vi "Method 5.vi"(11 "Test Interface in":refnum<class "Test Interface.lvclass">) -> (3 "Test Interface out":refnum<class "Test Interface.lvclass">)   [LabVIEW 2023, in "Test Interface.lvlib" / "Test Interface.lvclass"]
doc: "My Method Description"
uses:
  Test Interface.lvclass
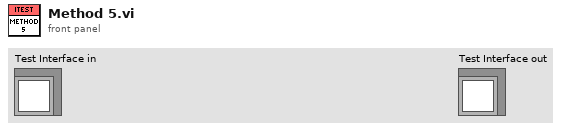
[diagram p1: front panel]
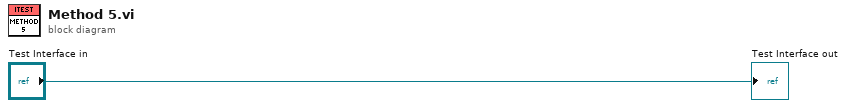
[diagram p0: block diagram]
diagram:
  "Test Interface out" <- "Test Interface in"
